vi "SelfTest.vi"(8 "error in (no error)":errorcluster, 11 "DigitalOutput_Simulation In":refnum<class "TesteractHAL_DigitalOutput_Simulation.lvclass">) -> (0 "error out":errorcluster, 1 "Self Test Result Message":string, 2 "Self Test Result Status":bool, 3 "DigitalOutput_Simulation Out":refnum<class "TesteractHAL_DigitalOutput_Simulation.lvclass">, 4 "Self Test Result Code":i32)   [LabVIEW 2017, in "TesteractHAL_DigitalOutput_Simulation.lvlib" / "TesteractHAL_DigitalOutput_Simulation.lvclass"]
uses:
  TesteractHAL_DigitalOutput_Simulation.lvclass
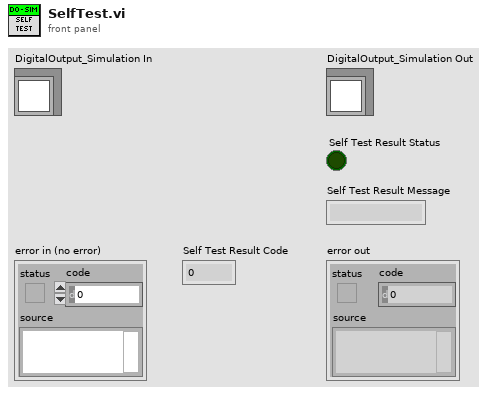
[diagram p1: front panel]
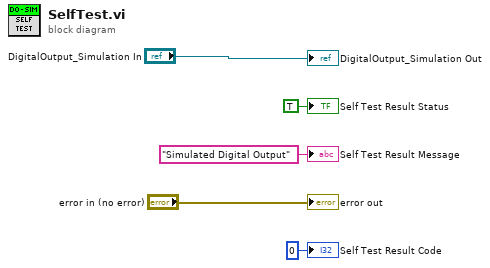
[diagram p0: block diagram]
diagram:
  "error out" <- "error in (no error)"
  "DigitalOutput_Simulation Out" <- "DigitalOutput_Simulation In"
  "Self Test Result Status" <- TRUE ("Self Test Result Status")
  "Self Test Result Code" <- 0 ("Self Test Result Code")
  "Self Test Result Message" <- "Simulated Digital Output" ("Self Test Result Message")
